vi "Update Pending Changes Enabled State.vi"(11 "UI Data in":refnum<class "Settings UI.lvclass">) -> (3 "UI Data out":refnum<class "Settings UI.lvclass">)   [LabVIEW 2020, in "Output Sequencer.lvlib" / "Settings UI.lvclass"]
uses:
  Settings UI.lvclass
  Settings UI.lvclass/Settings UI.ctl
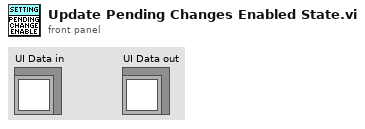
[diagram p1: front panel]
types:
  T1 = enum8{"Enabled", "Disabled", "Disabled and Grayed Out"}
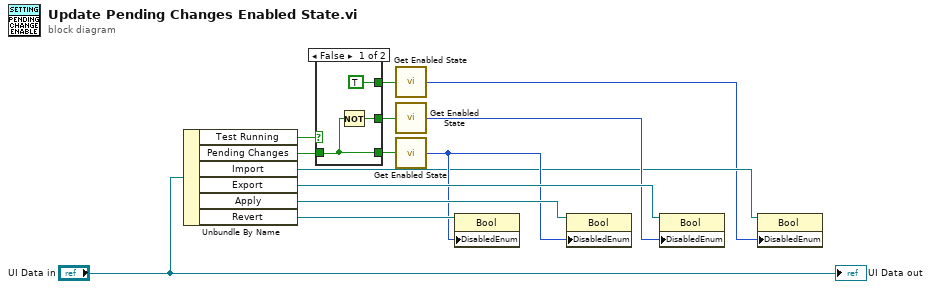
[diagram p0: block diagram]
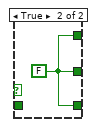
[diagram p2: hidden frame]
diagram:
  n1 = Unbundle By Name("UI Data in") -> ("Test Running"=w5:bool, "Pending Changes"=w7:bool, "Import"=w4:refnum<vi>, "Export"=w10:refnum<vi>, "Apply"=w11:refnum<vi>, "Revert"=w12:refnum<vi>)
  n2 = case shown="False" w5 {
    tunnel: [w16 w17] -> w3
    tunnel: w7 -> [w15 _]
    tunnel: [w15 w17] -> w6
    tunnel: [TRUE w17] -> w2
    frame False {
      n3 = Not(x=w15) -> (.not. x?=w16:bool)
    }
    frame True {
      w17 = FALSE
    }
  }
  n4 = call "Get Enabled State.vi"("Enabled?"=w2) -> ("State"=w1:T1)
  n5 = call "Get Enabled State.vi"("Enabled?"=w3) -> ("State"=w8:T1)
  n6 = call "Get Enabled State.vi"("Enabled?"=w6) -> ("State"=w9:T1)
  n7 = property class="Bool"(reference=w12, "DisabledEnum"=w9) -> ()  [unwired: 1 in, 2 out]
  n8 = property class="Bool"(reference=w11, "DisabledEnum"=w9) -> ()  [unwired: 1 in, 2 out]
  n9 = property class="Bool"(reference=w10, "DisabledEnum"=w8) -> ()  [unwired: 1 in, 2 out]
  n10 = property class="Bool"(reference=w4, "DisabledEnum"=w1) -> ()  [unwired: 1 in, 2 out]
  "UI Data out" <- "UI Data in"
